vi "0812_Controle_FMS.vi"() -> ()   [LabVIEW 2017]
uses:
  <vilib>/myRIO/Instrument Drivers/Onboard IO/PWM/typedefs/PWM Reference.ctl
  <vilib>/myRIO/Common/Instrument Driver Framework/Utilities/typedefs/myRIO Generic Hardware Reference.ctl
  <vilib>/myRIO/Common/Instrument Driver Framework/Utilities/typedefs/Hardware Version Enum.ctl
  <vilib>/myRIO/Common/Instrument Driver Framework/Utilities/typedefs/myRIO v1.0 Reference.ctl
  <vilib>/myRIO/Common/Instrument Driver Framework/Utilities/typedefs/Generic FPGA Reference.ctl
  <vilib>/myRIO/Common/Instrument Driver Framework/myRIO v1.0/PWM/typedefs/PWM Channels Enum.ctl
  <vilib>/myRIO/Instrument Drivers/Onboard IO/PWM/typedefs/PWM Configuration.ctl
  <vilib>/userdefined/High Color/nirio_resource_hc.ctl
  <vilib>/myRIO/Common/Instrument Driver Framework/myRIO v1.0/PWM/vis/myRIO v1.1 Open PWM.vi
  <vilib>/myRIO/Common/Instrument Driver Framework/Utilities/vis/Validate Channels.vi
  <vilib>/myRIO/Common/Instrument Driver Framework/myRIO v1.0/PWM/vis/myRIO v1.0 Reserve PWM.vi
  <vilib>/myRIO/Instrument Drivers/Onboard IO/PWM/vis/Set Duty Cycle and Frequency.vi
  <vilib>/myRIO/Common/Instrument Driver Framework/myRIO v1.0/PWM/vis/myRIO v1.0 Close PWM.vi
  <vilib>/myRIO/Common/Instrument Driver Framework/myRIO v1.0/PWM/vis/myRIO v1.0 Build MUX Configuration PWM.vi
  <vilib>/myRIO/Common/Instrument Driver Framework/myRIO v1.0/Resource Manager/vis/myRIO v1.0 Reserve Channel List.vi
  <vilib>/myRIO/Common/Instrument Driver Framework/myRIO v1.0/PWM/vis/myRIO v1.0 Unreserve PWM.vi
  <vilib>/myRIO/Common/Instrument Driver Framework/myRIO v1.0/Resource Manager/vis/myRIO v1.0 Create Configuration List.vi
  <vilib>/myRIO/Common/Instrument Driver Framework/myRIO v1.0/Resource Manager/vis/myRIO v1.0 Reserve Channel.vi
  <vilib>/myRIO/Common/Instrument Driver Framework/myRIO v1.0/Resource Manager/vis/myRIO v1.0 Unreserve Channel.vi
  <vilib>/myRIO/Common/Instrument Driver Framework/myRIO v1.0/Resource Manager/vis/myRIO v1.0 Unreserve Channel List.vi
  <vilib>/myRIO/Common/Instrument Driver Framework/myRIO v1.0/Resource Manager/vis/myRIO v1.0 Build Mutex Name.vi
  <vilib>/Utility/VariantDataType/GetNumericInfo.vi
  <vilib>/Utility/error.llb/Error Cluster From Error Code.vi
  <vilib>/myRIO/Common/Instrument Driver Framework/myRIO v1.0/myRIO v1.1 Open.vi
  <vilib>/myRIO/Common/Instrument Driver Framework/Utilities/vis/IO Manager.vi
  <vilib>/myRIO/Common/Instrument Driver Framework/Utilities/vis/Configuration Manager.vi
  <vilib>/myRIO/Common/Instrument Driver Framework/myRIO v1.0/Resource Manager/vis/myRIO v1.0 Configure IO.vi
  <vilib>/myRIO/Common/Instrument Driver Framework/myRIO v1.0/myRIO v1.0 Close.vi
  <vilib>/myRIO/Common/Instrument Driver Framework/myRIO v1.0/PWM/vis/myRIO v1.0 Write PWM.vi
  <vilib>/myRIO/Common/Instrument Driver Framework/myRIO v1.0/PWM/vis/myRIO v1.0 Shutdown PWM.vi
  <vilib>/myRIO/Instrument Drivers/Onboard IO/PWM/vis/myRIO PWM Open.xnode
  <vilib>/myRIO/Instrument Drivers/Onboard IO/PWM/PWM.lvlib
panel:
  out "ms":u32
  in  "Stop conveyor":bool=TRUE
  in  "Conveyor speed (mm/s)":dbl(slide)=200.0 step=1.0 scale=0.0..350.0
  in  "Actuator":bool
  in  "Stop":bool
  out "Position":dbl[](array[knob]) scale=0.0..200.0
  out "error out":errorcluster
  in  "error in (no error)":errorcluster
  in  "ms to wait (braço)":u32=5
  # "Range: 0,025 - 0,125\n\n3° = 0,00125\n\nLink 1 - (0,00125/3)x + 0,1\n0,125 -> 60°\n0,1 -> 0°\n0,0625 -> -90\n0,025 -> -180°\n\nLink 2 - -(0,00125/3)x + 0,1\n0,025 -> 180°\n0,0625 -> 90°\n0,1 -> 0°\n0,125 -> -60°\n\nLink 3 - (0,00125/3)x + 0,025\n0,125 -> 240°\n0,105 -> 180° \n0,63 -> 90°\n0,025 -> 0°\n\n9° = 0,05\n\nLink 5 - (0,005/9)x + 0,075\n0,125 -> 90°\n0,075 -> 0°\n0,025 ->-90°"
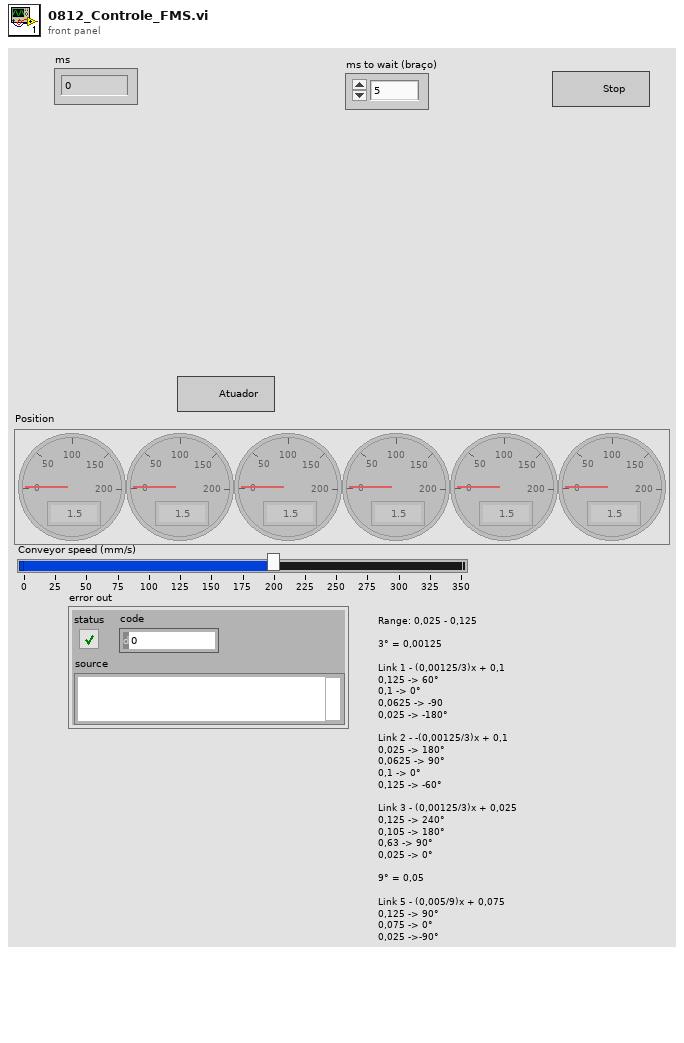
[diagram p1: front panel]
types:
  T1 = typedef "nirio_resource_hc.ctl" = tag
  T2 = typedef "Hardware Version Enum.ctl" = enum16{"Unknown", "myRIO-1900", "myRIO-1950", "roboRIO", "NI ELVIS RIO CM"}
  T3 = typedef "PWM.lvlib/PWM Reference.ctl" = cluster{"myRIO Reference":T4, "PWM Channels Enum":T7, "PWM Configuration":T8}
  T4 = typedef "myRIO Generic Hardware Reference.ctl" = cluster{"myRIO Model":T2, "myRIO Hardware Reference":T5}
  T5 = typedef "myRIO v1.0 Reference.ctl" = cluster{"Generic FPGA Reference":T6, "Allow multiple opens":bool}
  T6 = typedef "Generic FPGA Reference.ctl" = refnum<k20>
  T7 = typedef "PWM Channels Enum.ctl" = enum16{"Not Connected", "C/PWM0", "C/PWM1", "A/PWM0", "A/PWM1", "A/PWM2", "B/PWM0", "B/PWM1", "B/PWM2", "PWM/PWM0", "PWM/PWM1", "PWM/PWM2", "PWM/PWM3", "PWM/PWM4", "PWM/PWM5", "PWM/PWM6", "PWM/PWM7", "PWM/PWM8", "PWM/PWM9"}
  T8 = typedef "PWM.lvlib/PWM Configuration.ctl" = cluster{"Frequency":dbl, "Duty Cycle":dbl}
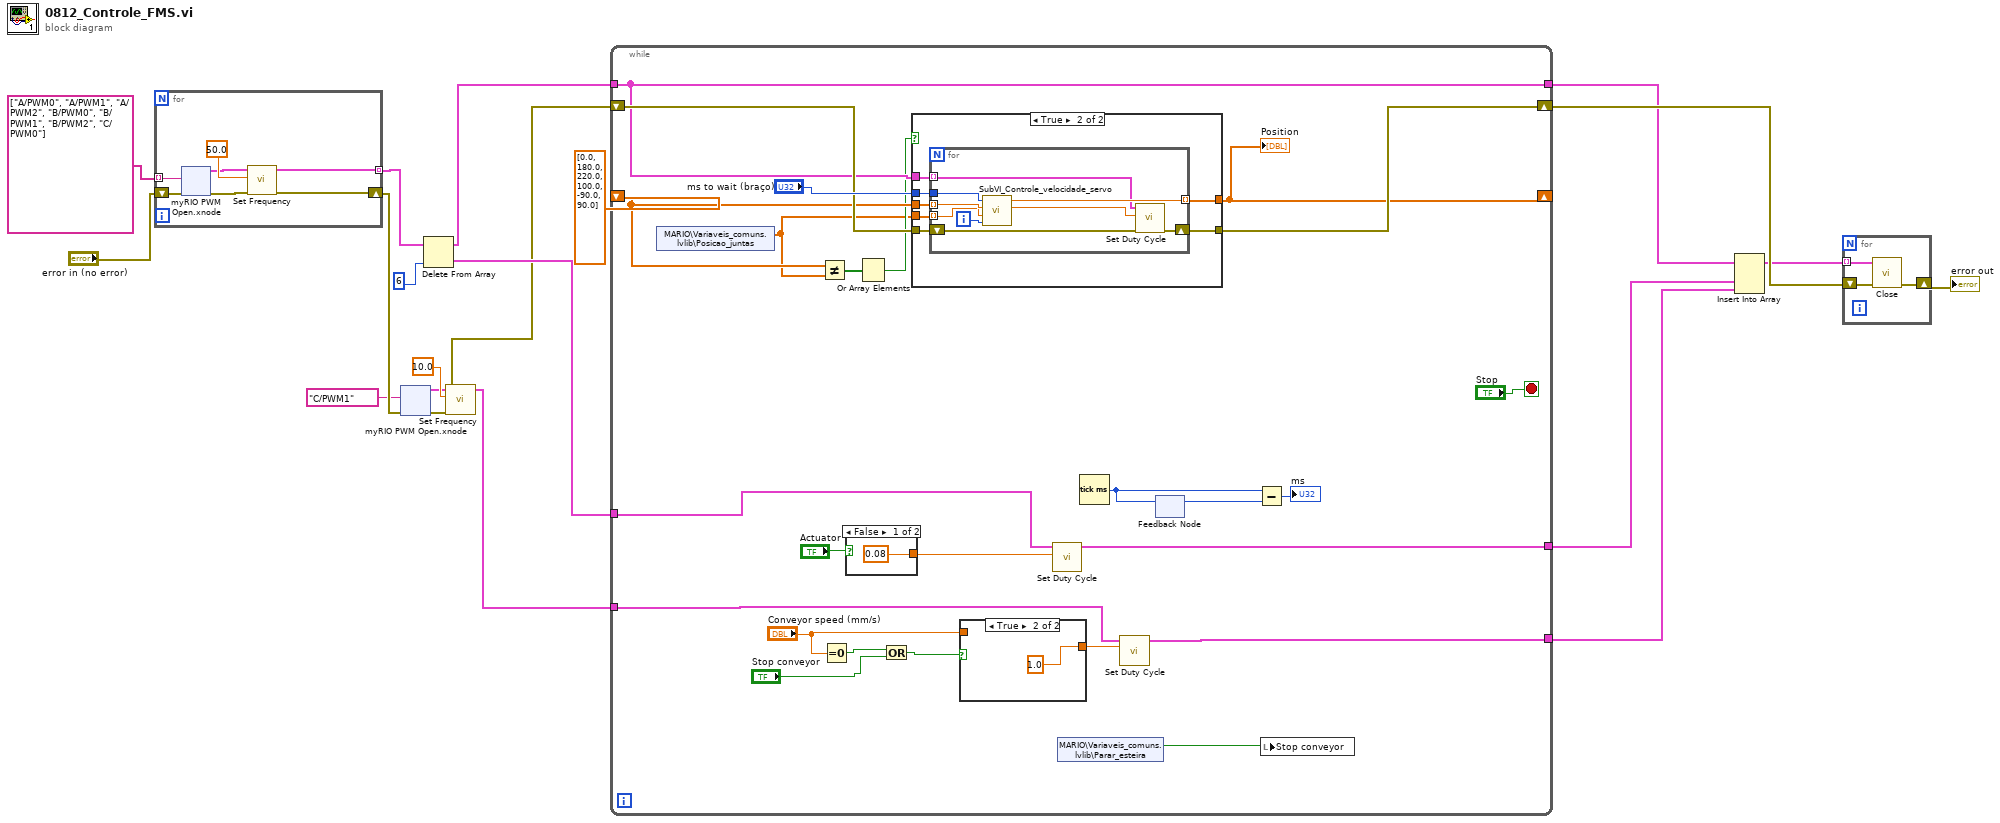
[diagram p0: block diagram]
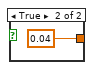
[diagram p3: hidden frame]
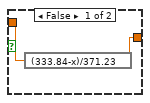
[diagram p4: hidden frame]
diagram:
  n1 = for {
    shift-right: [w21] -> w10
    shift-left: "error in (no error)" -> [w26]
    tunnel: tag[] ["A/PWM0", "A/PWM1", "A/PWM2", "B/PWM0", "B/PWM1", "B/PWM2", "C/PWM0"] -> [w27] mode=indexing
    tunnel: [w22] -> w7 mode=indexing
    n2 = xnode "myRIO PWM Open.xnode"("error in (no error)"=w26, "Channel Name"=w27) -> ("error out"=w24:errorcluster, "PWM Ref Out"=w23:T3)  [unwired: 1 in]
    n3 = call <vilib>:"Set Frequency.vi"("error in (no error)"=w24, "Frequency [Hz]"=50.0, "PWM Ref In"=w23) -> ("error out"=w21:errorcluster, "PWM Ref Out"=w22:T3)  [unwired: 6 in]
  }
  n4 = xnode "myRIO PWM Open.xnode"("error in (no error)"=w10, "Channel Name"=tag "C/PWM1") -> ("error out"=w11:errorcluster, "PWM Ref Out"=w12:T3)  [unwired: 1 in]
  n5 = Delete From Array(array=w7, index=6) -> (deleted portion=w4:T3, array with subset deleted=w5:T3[])  [unwired: 1 in]
  n6 = call <vilib>:"Set Frequency.vi"("error in (no error)"=w11, "Frequency [Hz]"=10.0, "PWM Ref In"=w12) -> ("error out"=w3:errorcluster, "PWM Ref Out"=w2:T3)  [unwired: 6 in]
  n7 = while {
    shift-right: [w66] -> w20
    shift-left: w3 -> [w67]
    shift-right: [w65] -> _
    shift-left: dbl[] [0.0, 180.0, 220.0, 100.0, -90.0, 90.0] -> [w51]
    tunnel: w5 -> [w64]
    tunnel: [w64] -> w17
    tunnel: w4 -> [w62]
    tunnel: [w60] -> w16
    tunnel: w2 -> [w58]
    tunnel: [w56] -> w14
    stop <- "Stop" stop-if-true
    n8 = shared-variable "MARIO\\Variaveis_comuns.lvlib\\Posicao_juntas"() -> (w44:dbl[])  [unwired: 1 in, 1 out]
    n9 = Not Equal?(x=w51, y=w44) -> (x != y?=w50:bool[])
    n10 = Equal To 0?(x="Conveyor speed (mm/s)") -> (x = 0?=w49:bool)
    n11 = case shown="False" "Actuator" {
      tunnel: [0.08 ("Duty Cycle Abert") 0.04 ("Duty Cycle Abert")] -> w61
      frame False {
      }
      frame True {
      }
    }
    n12 = Or Array Elements(Boolean array=w50) -> (logical OR=w48:bool)
    n13 = Or(x=w49, y="Stop conveyor") -> (x .or. y?=w55:bool)
    n14 = case shown="True" w48 {
      tunnel: "ms to wait (braço)" -> [_ w77]
      tunnel: w44 -> [_ w76]
      tunnel: w67 -> [w70 w75]
      tunnel: [w70 w74] -> w66
      tunnel: [w69 w73] -> w65
      tunnel: w64 -> [_ w72]
      tunnel: w51 -> [w69 w71]
      frame False {
      }
      frame True {
        n15 = for {
          tunnel: w77 -> [w86]
          tunnel: w72 -> [w81] mode=indexing
          tunnel: w76 -> [w79] mode=indexing
          tunnel: w71 -> [w80] mode=indexing
          shift-right: [w82] -> w74
          shift-left: w75 -> [w83]
          tunnel: [w85] -> w73 mode=indexing
          i -> [w78]
          n16 = call "SubVI_Controle_velocidade_servo.vi"("Link"=w78, "Posição Desejada"=w79, "Posição"=w80, "milliseconds to wait"=w86) -> ("Duty Cycle"=w84:dbl, "Posição"=w85:dbl)  [unwired: 6 in]
          n17 = call <vilib>:"Set Duty Cycle.vi"("error in (no error)"=w83, "Duty Cycle"=w84, "PWM Ref In"=w81) -> ("error out"=w82:errorcluster)  [unwired: 6 in, 1 out]
        }
      }
    }
    "Position" <- w65
    n18 = case shown="True" w55 {
      tunnel: [w89 1.0] -> w57
      tunnel: "Conveyor speed (mm/s)" -> [w90 _]
      frame False {
        n19 = expression code="(333.84-x)/371.23"(w90) -> (w89:dbl)
      }
      frame True {
      }
    }
    n20 = call <vilib>:"Set Duty Cycle.vi"("Duty Cycle"=w61, "PWM Ref In"=w62) -> ("PWM Ref Out"=w60:T3)  [unwired: 7 in, 1 out]
    n21 = shared-variable "MARIO\\Variaveis_comuns.lvlib\\Parar_esteira"() -> (w47:bool)  [unwired: 1 in, 1 out]
    n22 = Tick Count (ms)() -> (millisecond timer value=w53:u32)
    n23 = call <vilib>:"Set Duty Cycle.vi"("Duty Cycle"=w57, "PWM Ref In"=w58) -> ("PWM Ref Out"=w56:T3)  [unwired: 7 in, 1 out]
    n24 = feedback-in #1(w53) -> ()
    n25 = feedback #1() -> (w52:u32)  [unwired: 1 in]
    n26 = Subtract(x=w53, y=w52) -> (x-y=→"ms":u32)
    n27 = local write "Stop conveyor"(w47) -> ()
  }
  n28 = Insert Into Array(array=w17, new element #1=w16, new element #2=w14) -> (w15:T3[])  [unwired: 1 in]
  n29 = for {
    tunnel: w15 -> [w94] mode=indexing
    shift-right: [w92] -> w19
    shift-left: w20 -> [w93]
    n30 = call <vilib>:"Close.vi"("error in (no error)"=w93, "PWM Ref In"=w94) -> ("error out"=w92:errorcluster)  [unwired: 9 in]
  }
  "error out" <- w19
